vi "VI Tree.vi"   [LabVIEW 2017, in "ADCMT7451_ADC.lvlib"]
doc: "This is the instrument driver for the <INSTRUMENT NAME>. The VI Tree displays all the user-callable VIs of the instrument driver in an organized table."
uses:
  ADCMT7451_ADC.lvlib
panel:
  # "(c) 2007 ADCMT ADC CORPORATION  ALL RIGHTS RESERVED."
  # "SEE DIAGRAM\nFOR VI TREE."
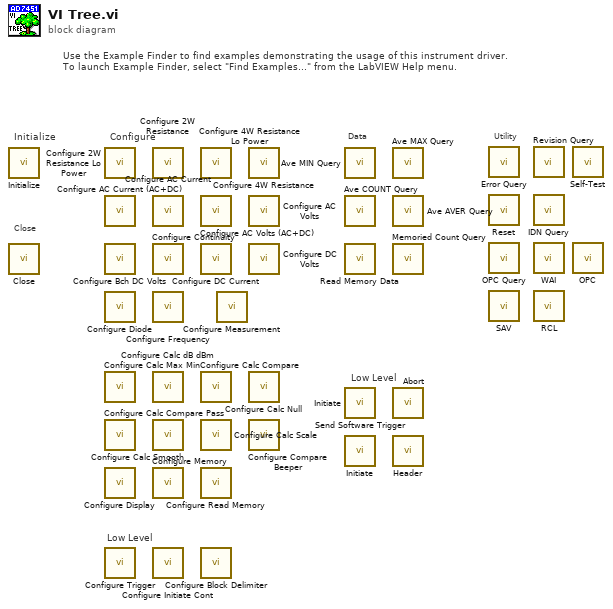
[diagram p0: block diagram]
diagram:
  # "Low Level"
  # "Low Level"
  # "Use the Example Finder to find examples demonstrating the usage of this instrument driver.\nTo launch Example Finder, select \"Find Examples...\" from the LabVIEW Help menu."
  # "Configure"
  # "Utility"
  # "Data"
  # "Close"
  # "Initialize"
  n1 = call "Initialize.vi"() -> ()  [unwired: 10 in, 2 out]
  n2 = call "Close.vi"() -> ()  [unwired: 11 in, 1 out]
  n3 = call "Configure 2W Resistance Lo Power.vi"() -> ()  [unwired: 18 in, 2 out]
  n4 = call "Configure AC Current (AC+DC).vi"() -> ()  [unwired: 18 in, 2 out]
  n5 = call "Configure Bch DC Volts.vi"() -> ()  [unwired: 18 in, 2 out]
  n6 = call "Configure Diode.vi"() -> ()  [unwired: 18 in, 2 out]
  n7 = call "Configure Calc Max Min.vi"() -> ()  [unwired: 10 in, 2 out]
  n8 = call "Configure Calc Compare Pass.vi"() -> ()  [unwired: 10 in, 2 out]
  n9 = call "Configure Display.vi"() -> ()  [unwired: 10 in, 2 out]
  n10 = call "Configure Trigger.vi"() -> ()  [unwired: 18 in, 2 out]
  n11 = call "Configure 2W Resistance.vi"() -> ()  [unwired: 18 in, 2 out]
  n12 = call "Configure AC Current.vi"() -> ()  [unwired: 18 in, 2 out]
  n13 = call "Configure Continuity.vi"() -> ()  [unwired: 18 in, 2 out]
  n14 = call "Configure Frequency.vi"() -> ()  [unwired: 18 in, 2 out]
  n15 = call "Configure Calc dB dBm.vi"() -> ()  [unwired: 10 in, 2 out]
  n16 = call "Configure Calc Smooth.vi"() -> ()  [unwired: 10 in, 2 out]
  n17 = call "Configure Memory.vi"() -> ()  [unwired: 10 in, 2 out]
  n18 = call "Configure Initiate Cont.vi"() -> ()  [unwired: 10 in, 2 out]
  n19 = call "Configure 4W Resistance Lo Power.vi"() -> ()  [unwired: 18 in, 2 out]
  n20 = call "Configure AC Volts (AC+DC).vi"() -> ()  [unwired: 18 in, 2 out]
  n21 = call "Configure DC Current.vi"() -> ()  [unwired: 18 in, 2 out]
  n22 = call "Configure Calc Compare.vi"() -> ()  [unwired: 9 in, 2 out]
  n23 = call "Configure Calc Scale.vi"() -> ()  [unwired: 10 in, 2 out]
  n24 = call "Configure Read Memory.vi"() -> ()  [unwired: 9 in, 3 out]
  n25 = call "Configure Block Delimiter.vi"() -> ()  [unwired: 10 in, 2 out]
  n26 = call-poly "Configure Measurement.vi"() -> ()  [unwired: 18 in, 2 out]
  n27 = call "Configure 4W Resistance.vi"() -> ()  [unwired: 18 in, 2 out]
  n28 = call "Configure AC Volts.vi"() -> ()  [unwired: 18 in, 2 out]
  n29 = call "Configure DC Volts.vi"() -> ()  [unwired: 18 in, 2 out]
  n30 = call "Configure Calc Null.vi"() -> ()  [unwired: 10 in, 2 out]
  n31 = call "Configure Compare Beeper.vi"() -> ()  [unwired: 10 in, 2 out]
  n32 = call "Ave MIN Query.vi"() -> ()  [unwired: 9 in, 3 out]
  n33 = call "Ave COUNT Query.vi"() -> ()  [unwired: 9 in, 3 out]
  n34 = call "Read Memory Data.vi"() -> ()  [unwired: 9 in, 3 out]
  n35 = call "Send Software Trigger.vi"() -> ()  [unwired: 10 in, 2 out]
  n36 = call "Initiate.vi"() -> ()  [unwired: 10 in, 2 out]
  n37 = call "Initiate.vi"() -> ()  [unwired: 10 in, 2 out]
  n38 = call "Ave MAX Query.vi"() -> ()  [unwired: 9 in, 3 out]
  n39 = call "Ave AVER Query.vi"() -> ()  [unwired: 9 in, 3 out]
  n40 = call "Memoried Count Query.vi"() -> ()  [unwired: 1 in]
  n41 = call "Abort.vi"() -> ()  [unwired: 10 in, 2 out]
  n42 = call "Header.vi"() -> ()  [unwired: 10 in, 2 out]
  n43 = call "Error Query.vi"() -> ()  [unwired: 8 in, 4 out]
  n44 = call "Reset.vi"() -> ()  [unwired: 10 in, 2 out]
  n45 = call "OPC Query.vi"() -> ()  [unwired: 9 in, 3 out]
  n46 = call "SAV.vi"() -> ()  [unwired: 9 in, 2 out]
  n47 = call "Revision Query.vi"() -> ()  [unwired: 8 in, 4 out]
  n48 = call "IDN Query.vi"() -> ()  [unwired: 9 in, 3 out]
  n49 = call "WAI.vi"() -> ()  [unwired: 10 in, 2 out]
  n50 = call "RCL.vi"() -> ()  [unwired: 9 in, 2 out]
  n51 = call "Self-Test.vi"() -> ()  [unwired: 8 in, 4 out]
  n52 = call "OPC.vi"() -> ()  [unwired: 10 in, 2 out]
